vi "split_cluster.vi"(8 "Clustering":i32[](array[numeric]), 10 "W":dbl[][](array[numeric]), 11 "STFT Spectrogram {X}":dbl[][](array[numeric])) -> (2 "N(number of Clusters)":i32, 3 "Splited_X(t)":dbl[][](array[numeric]))   [LabVIEW 2014]
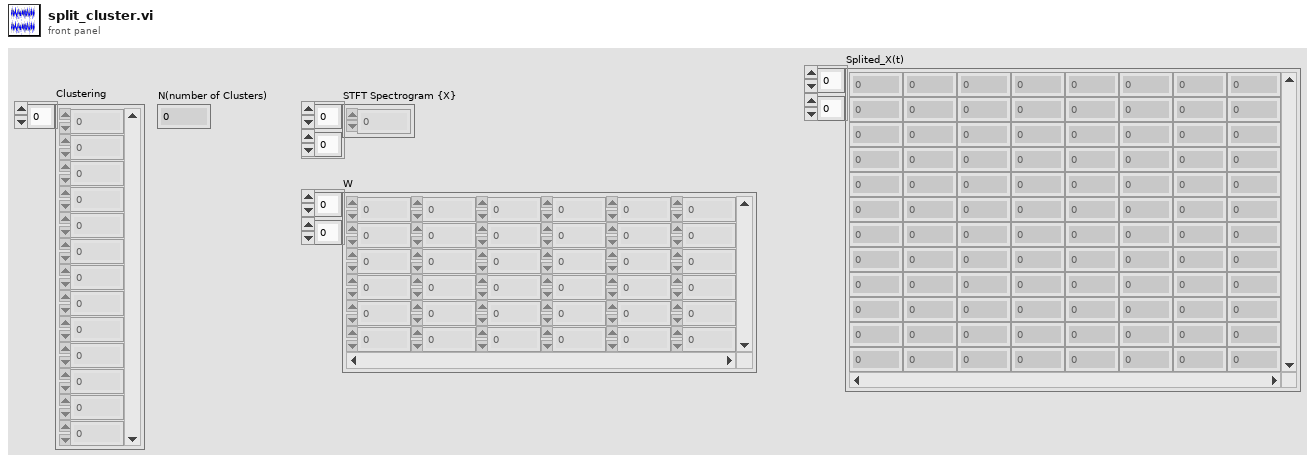
[diagram p1: front panel]
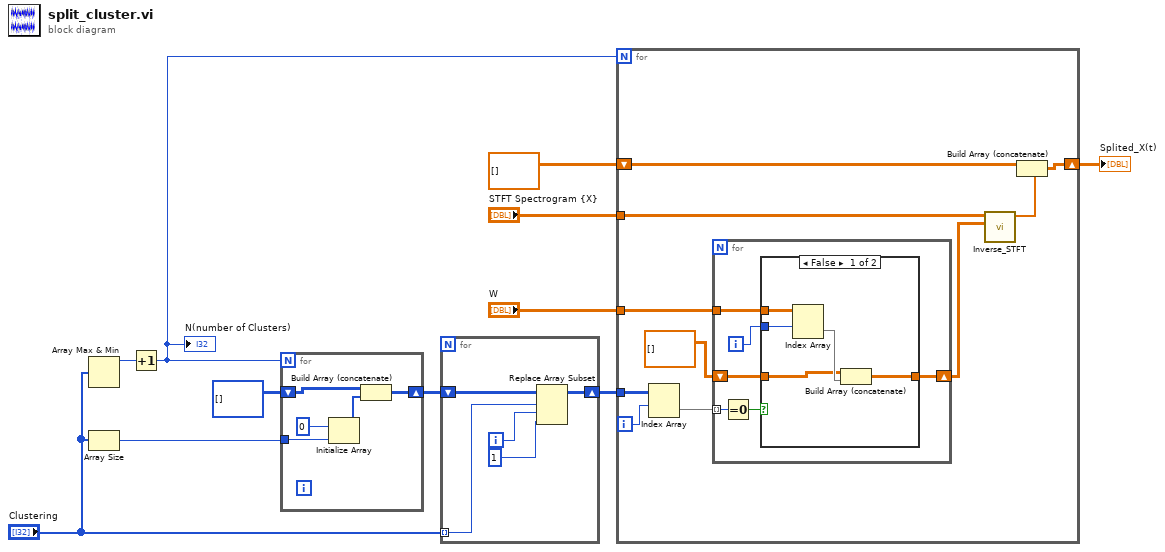
[diagram p0: block diagram]
diagram:
  n1 = Array Max & Min(array="Clustering") -> (max value=w11:i32)  [unwired: 3 out]
  n2 = Array Size(array="Clustering") -> (size(s)=w10:i32)
  n3 = Increment(x=w11) -> (x+1=w6:i32)
  "N(number of Clusters)" <- w6
  n4 = for {
    N: w6 -> [_]
    tunnel: w10 -> [w12]
    shift-right: [w15] -> w8
    shift-left: i32[][] [] -> [w14]
    n5 = Initialize Array(0 ("dimension size"), w12) -> (w16:i32[])
    n6 = Build Array (concatenate)(w14, w16) -> (w15:i32[][])
  }
  n7 = for {
    shift-right: [w17] -> w4
    shift-left: w8 -> [w21]
    tunnel: "Clustering" -> [w20] mode=indexing
    i -> [w19]
    n8 = Replace Array Subset(array=w21, new element=1 ("new element/subarray"), index (row)=w20, index (col)=w19) -> (w17:i32[][])
  }
  n9 = for {
    N: w6 -> [_]
    tunnel: "W" -> [w27]
    tunnel: w4 -> [w30]
    tunnel: "STFT Spectrogram {X}" -> [w31]
    shift-right: [w24] -> w1
    shift-left: dbl[][] [] -> [w23]
    i -> [w29]
    n10 = Index Array(array=w30, index (row)=w29) -> (element=w28:i32[])  [unwired: 1 in]
    n11 = for {
      tunnel: w28 -> [w37] mode=indexing
      tunnel: w27 -> [w35]
      shift-right: [w33] -> w22
      shift-left: dbl[][] [] -> [w32]
      i -> [w34]
      n12 = Equal To 0?(x=w37) -> (x = 0?=w36:bool)
      n13 = case shown="False" w36 {
        tunnel: w35 -> [w42 _]
        tunnel: w34 -> [w41 _]
        tunnel: [w39 w43] -> w33
        tunnel: w32 -> [w38 w43]
        frame False {
          n14 = Index Array(array=w42, index (row)=w41) -> (element=w40:dbl[])  [unwired: 1 in]
          n15 = Build Array (concatenate)(w38, w40) -> (w39:dbl[][])
        }
        frame True {
        }
      }
    }
    n16 = call "Inverse_STFT.vi"("W"=w22, "STFT Spectrogram {X}"=w31) -> ("Inverse_STFT"=w25:dbl[])  [unwired: 9 in]
    n17 = Build Array (concatenate)(w23, w25) -> (w24:dbl[][])
  }
  "Splited_X(t)" <- w1
